vi "Set message.vi"(10 "WampMessage MsgPack":refnum<class "WampMessage MsgPack.lvclass">, 11 "IMsgPackMessageHandler in":refnum<class "IMsgPackMessageHandler.lvclass">) -> (3 "IMsgPackMessageHandler out":refnum<class "IMsgPackMessageHandler.lvclass">)   [LabVIEW 2020, in "wamplv.lvlib" / "IMsgPackMessageHandler.lvclass"]
uses:
  IMsgPackMessageHandler.lvclass
  SerialisedMessages/MsgPackMessage/WampMessage MsgPack.lvclass
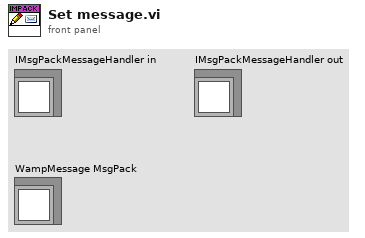
[diagram p1: front panel]
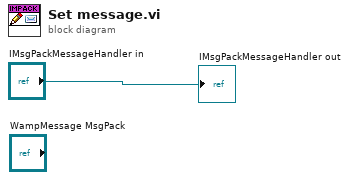
[diagram p0: block diagram]
diagram:
  "IMsgPackMessageHandler out" <- "IMsgPackMessageHandler in"
